vi "Demo.vi"() -> ()   [LabVIEW 2020]
uses:
  <vilib>/vision/driver/NI_Vision_Acquisition_Software.lvlib
  <vilib>/userdefined/High Color/IMAQdx.ctl
panel:
  in  "Acquisition Mode":enum16{"Grab", "Snap"}(ring)
  out "Measurements":T1(plugin-control)
  out "Error Out":errorcluster
  out "# Iter":i32
  in  "Start":bool
  out "Image":T1(plugin-control)
  in  "Stop":bool
  out "Template":T1(plugin-control)
  in  "Inspection Part":enum32{"P1", "P2", "P3"}(tab)
  out "P1 Matches":i32
  out "Top Inner":dbl format="%#_5g"
  out "Top Outer":dbl format="%#_5g"
  out "Outer Ring":dbl format="%#_5g"
  out "P1 Status":bool caption="Status"
  out "Top Outer Status":bool
  out "Outer Ring Status":bool
  out "Top Inner Status":bool
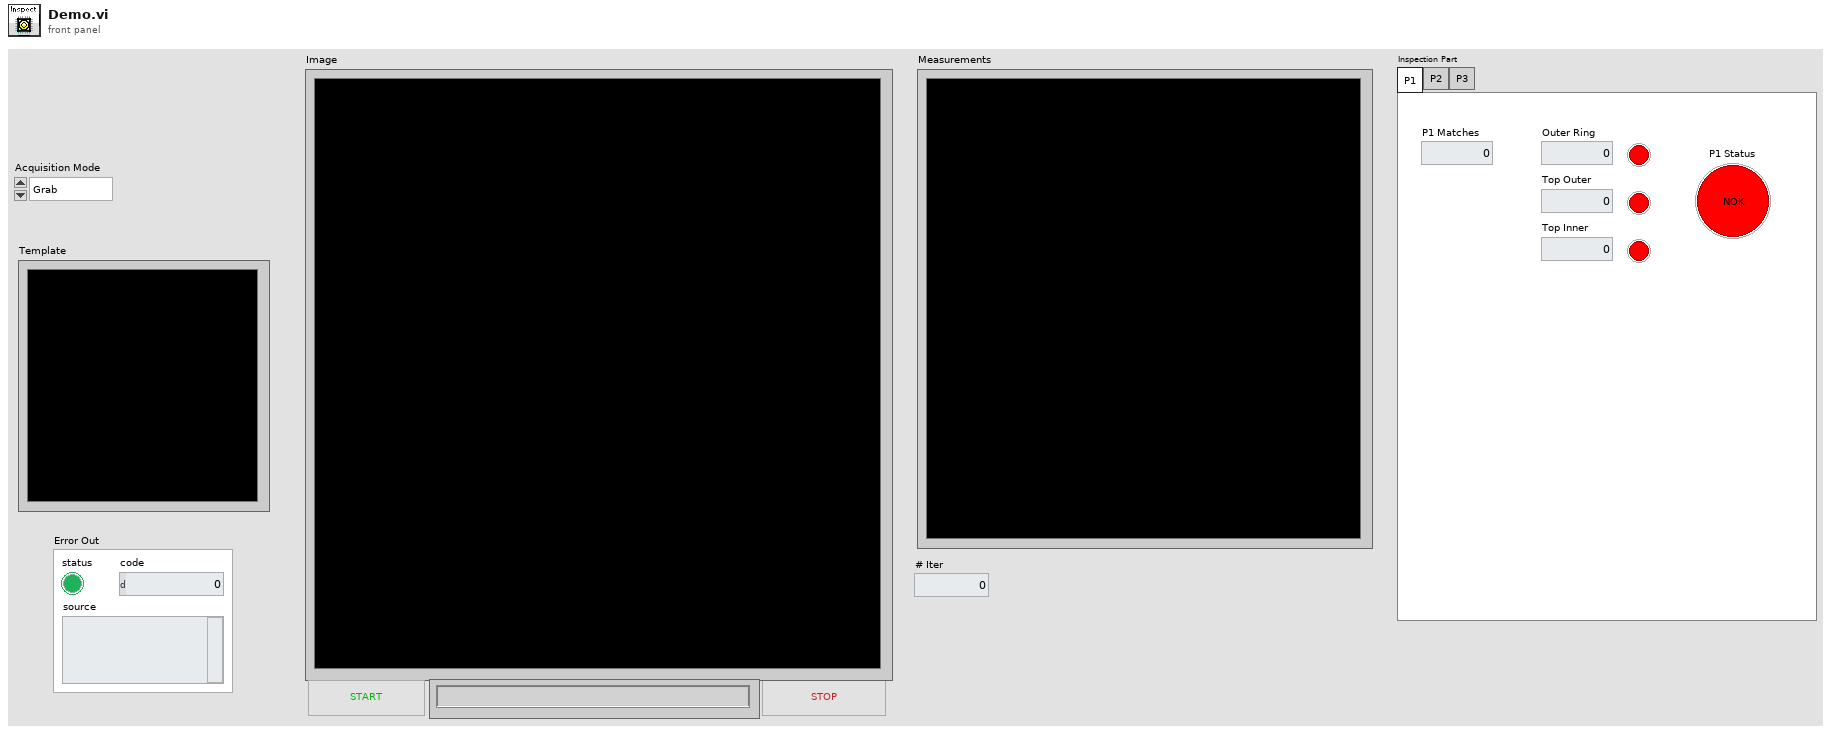
[diagram p1: front panel]
types:
  T1 = typedef "IMAQ Image.ctl" = refnum<image>
  T2 = typedef "IMAQdx.ctl" = refnum<k21>
  T3 = cluster{"Desired Font (Application)":enum16{"User-specified Font", "Application Font", "System Font", "Dialog Font"}, "[User-specified Font]":cluster{"Font Name":string, "Size":i16, "Strikeout?":bool, "Italic?":bool, "Underline?":bool, "Outline?":bool, "Shadow?":bool, "Bold?":bool, "Rotation Angle":dbl}, "Horizontal Alignment":i16, "Vertical Alignment":i16}
  T4 = typedef "Image Type" = u32
  T5 = typedef "ROI Descriptor" = cluster{"Global Rectangle":i32[], "Contours":cluster{"ID":enum32{"External", "Internal"}, "Type":u32, "Coordinates":i32[]}[]}
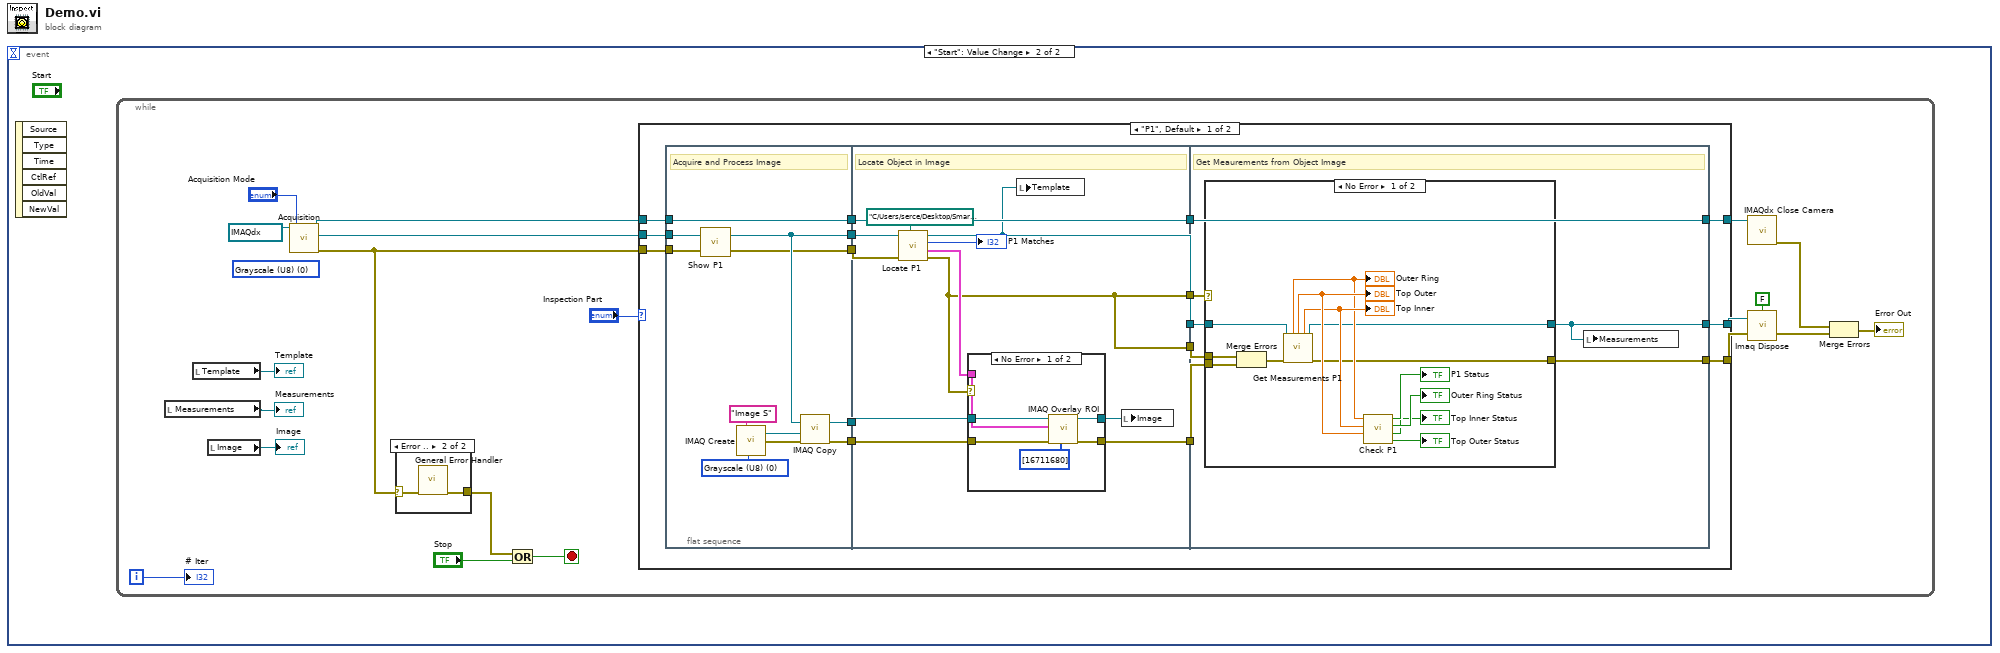
[diagram p0: block diagram]
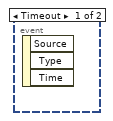
[diagram p2: hidden frame]
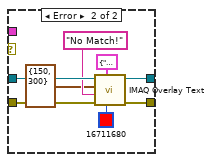
[diagram p4: hidden frame]
diagram:
  n1 = event shown="[1] \"Start\": Value Change" {
    selector: _ -> [_ _]
    dyn-events: _ -> [_ _]
    timeout: _ -> [_ _]
    event Timeout {
      n2 = event-data() -> ()  [unwired: 1 in, 3 out]
    }
    event "Start": Value Change {
      n3 = event-data() -> ()  [unwired: 1 in, 6 out]
      n4 = while {
        i -> [w20]
        stop <- w6 stop-if-true
        (unwired) T4 0 items=["Grayscale (U8)", "Grayscale (I16)", "Grayscale (SGL)", "Complex (CSG)", "RGB (U32)", "HSL (U32)", "RGB (U64)", "Grayscale (U16)"] ("Image Type")
        n5 = local read "Measurements"() -> (→"Measurements":T1)
        n6 = local read "Template"() -> (→"Template":T1)
        n7 = local read "Image"() -> (→"Image":T1)
        n8 = call "Acquisition.vi"("Mode"="Acquisition Mode", "Session In"=T2 "cam3") -> ("Error Out"=w2:errorcluster, "Image Out"=w9:T1, "IMAQdx Session Out"=w8:T2)  [unwired: 7 in]
        n9 = case shown="Error .." w2 {
          selector: w2 -> [w21 w23]
          tunnel: [w21 w22] -> w1
          frame No Error {
          }
          frame Error {
            n10 = call <vilib>:"General Error Handler.vi"("error in (no error)"=w23) -> ("error out"=w22:errorcluster)  [unwired: 10 in, 4 out]
          }
        }
        n11 = Or(x=w1, y="Stop") -> (x .or. y?=w6:bool)
        n12 = case shown="\"P1\", Default" "Inspection Part" {
          tunnel: w9 -> [w30 _]
          tunnel: w2 -> [w29 _]
          tunnel: w8 -> [w28 _]
          tunnel: [w27 _] -> w5
          tunnel: [w26 _] -> w4
          tunnel: [w25 _] -> w3
          frame "P1", Default {
            n13 = flat-sequence {
              tunnel: [w40] -> w39
              tunnel: [w46] -> w38
              tunnel: [w45] -> w37
              tunnel: [w44] -> w36
              tunnel: [w43] -> w35
              tunnel: w30 -> [w42]
              tunnel: w29 -> [w41]
              tunnel: w28 -> [w40]
              tunnel: w39 -> [w59]
              tunnel: [w54] -> w34
              tunnel: [w52] -> w33
              tunnel: [w62] -> w32
              tunnel: w38 -> [w61]
              tunnel: w37 -> [w60]
              tunnel: w36 -> [w58]
              tunnel: w35 -> [w57]
              tunnel: [w59] -> w31
              tunnel: [w52] -> w24
              tunnel: w34 -> [w81]
              tunnel: w33 -> [w83]
              tunnel: w32 -> [w82]
              tunnel: w31 -> [w80]
              tunnel: [w80] -> w27
              tunnel: [w79] -> w26
              tunnel: [w77] -> w25
              tunnel: w24 -> [w78]
              frame #0 {
                w49 = T4 0 items=["Grayscale (U8)", "Grayscale (I16)", "Grayscale (SGL)", "Complex (CSG)", "RGB (U32)", "HSL (U32)", "RGB (U64)", "Grayscale (U16)"] ("Image Type")
                # "Acquire and Process Image"
                n14 = call "Show P1.vi"("Error In"=w41, "Image In"=w42) -> ("Error Out"=w43:errorcluster, "Image Out"=w44:T1)
                n15 = call "IMAQ Create"("Image Name"="Image S", "Image Type"=w49) -> ("New Image"=w48:T1, "error out"=w47:errorcluster)  [unwired: 3 in]
                n16 = call "IMAQ Copy"("error in (no error)"=w47, "Image Dst"=w48, "Image Src"=w44) -> ("error out"=w45:errorcluster, "Image Dst Out"=w46:T1)  [unwired: 3 in]
              }
              frame #1 {
                # "Locate Object in Image"
                n17 = call "Locate P1.vi"("Template File Path"=path "C:/Users/serce/Desktop/Smart Vision System Testbench/P1 Pattern.png", "Error In"=w57, "Image In"=w58) -> ("Error Out"=w52:errorcluster, "Number of Matches (Pattern Matching)"=→"P1 Matches":i32, "Object Out"=w54:T1, "ROI Descriptor out"=w55:T5)  [unwired: 3 in]
                n18 = case shown="No Error" w52 {
                  tunnel: [w67 w75] -> w62
                  tunnel: w61 -> [w66 w73]
                  tunnel: w60 -> [w65 w76]
                  tunnel: w55 -> [w64 _]
                  tunnel: [w63 w74] -> w51
                  frame No Error {
                    n19 = call "IMAQ Overlay ROI"("Colors (Green)"=u32[] [16711680], "error in (no error)"=w65, "ROI Descriptor"=w64, "Image"=w66) -> ("error out"=w67:errorcluster, "Image Out"=w63:T1)  [unwired: 6 in]
                  }
                  frame Error {
                    n20 = call "IMAQ Overlay Text"("Text Color (black)"=u32 16711680, "Font, Size & Style"=T3 {"Desired Font (Application)"=enum."User-specified Font", "[User-specified Font]"={"Font Name"="System Font", "Size"=152, "Strikeout?"=FALSE, "Italic?"=FALSE, "Underline?"=FALSE, "Outline?"=TRUE, "Shadow?"=FALSE, "Bold?"=FALSE, "Rotation Angle"=0.0}, "Horizontal Alignment"=0, "Vertical Alignment"=0}, "error in (no error)"=w76, "String"="No Match!", "Origin"=cluster{"X":i32, "Y":i32} {"X"=150, "Y"=300}, "Image"=w73) -> ("error out"=w75:errorcluster, "Image Out"=w74:T1)  [unwired: 4 in]
                  }
                }
                n21 = local write "Template"(w54) -> ()
                n22 = local write "Image"(w51) -> ()
              }
              frame #2 {
                # "Get Meaurements from Object Image"
                n23 = case shown="No Error" w78 {
                  selector: w78 -> [_ w97]
                  tunnel: w83 -> [w96 _]
                  tunnel: w82 -> [w95 _]
                  tunnel: w81 -> [w93 w98]
                  tunnel: [w85 w97] -> w79
                  tunnel: [w84 w98] -> w77
                  frame No Error {
                    n24 = Merge Errors(w96, w95) -> (w94:errorcluster)
                    n25 = call "Get Measurements P1.vi"("Image In"=w93, "Error In"=w94) -> ("Outer Ring"=w86:sgl, "Top Outer"=w92:sgl, "Top Inner"=w91:sgl, "Image Out"=w84:T1, "Error Out"=w85:errorcluster)  [unwired: 8 in, 1 out]
                    "Outer Ring" <- w86
                    "Top Outer" <- w92
                    "Top Inner" <- w91
                    n26 = call "Check P1.vi"("Top Outer"=w92, "Top Inner"=w91, "Outer Ring"=w86) -> ("Top Outer Status"=→"Top Outer Status":bool, "Top Inner Status"=→"Top Inner Status":bool, "Outer Ring Status"=→"Outer Ring Status":bool, "P1 Status"=→"P1 Status":bool)  [unwired: 1 in]
                  }
                  frame Error {
                  }
                }
                n27 = local write "Measurements"(w77) -> ()
              }
            }
          }
          frame "P2" {
          }
        }
        n28 = call <vilib>:"IMAQdx Close Camera.vi"("Session In"=w5) -> ("error out"=w14:errorcluster)  [unwired: 10 in]
        n29 = call "Imaq Dispose"("All Images? (No)"=FALSE, "Image"=w3, "error in (no error)"=w4) -> ("error out"=w13:errorcluster)  [unwired: 3 in]
        n30 = Merge Errors(w14, w13) -> (→"Error Out":errorcluster)
        "# Iter" <- w20
      }
    }
  }
